vi "Pack Mag Dev Msg.vi"(11 "Compass Mag Dev":dbl) -> (3 "Set Mag Dev Message out":refnum<class "Set Mag Dev Message.lvclass">)   [LabVIEW 2015, in "Compass Instrument.lvlib"]
uses:
  Compass Instrument.lvlib
  Libraries/RDS Child Messages/Compass/Set Mag Dev Message.lvclass
  Libraries/RDS Framework/RDS Message ID.ctl
  Libraries/RDS Framework/RDS Message Class/RDS Message.lvclass/RDS Message.ctl
  Libraries/RDS Child Messages/Compass/Set Mag Dev Message.lvclass/Set Mag Dev Message.ctl
  Libraries/RDS Framework/RDS Message Class/RDS Message.lvclass
  Libraries/RDS Child Messages/RDS Child Messages.lvlib
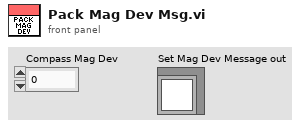
[diagram p1: front panel]
types:
  T1 = typedef "RDS Child Messages.lvlib/RDS Message ID.ctl" = enum16{"RDS Hello World", "String Message", "AIP_Status", "AIP_Command", "GPS_Data", "MCB_Command", "MCB_Status", "Compass_Data", "Depth_Data", "Battery_Data", "Contoller_State", "Set_Mag_Dev", "BTB_Shutdown", "State_Sample_Request", "State_Sample", "PID_Gains_Set", "Helm_Limiter_Set", "Helm_Heading_Command", "Helm_Steering_Command", "Helm_Status", "Controller_Message", "AIP_Set_Min_Depth", "Mission_Controller_State", "Mission_Upload", "Mission_Set_Op_and_Run", "Mission_Settings_Set"}
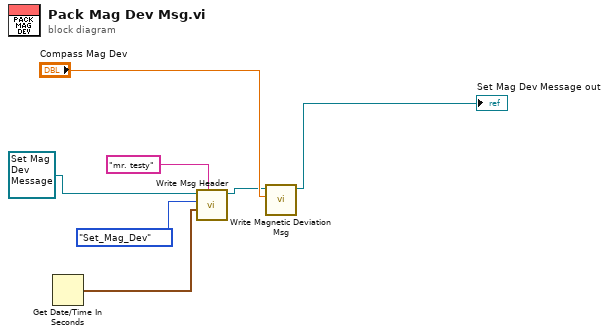
[diagram p0: block diagram]
diagram:
  n1 = Get Date/Time In Seconds() -> (seconds since 1Jan1904=w2:timestamp)
  n2 = call "Write Msg Header.vi"("Sender Name"="mr. testy", "Time Stamp"=w2, "Msg ID"=RDS_Message_ID."Set_Mag_Dev", "RDS Message in"=refnum<class "Set Mag Dev Message.lvclass"> refnum ("RDS Child Messages.lvlib:Set Mag Dev Message.lvclass")) -> ("RDS Message out"=w5:refnum<class "Set Mag Dev Message.lvclass">)  [unwired: 6 in, 1 out]
  n3 = call "Write Magnetic Deviation Msg.vi"("Magnetic Deviation"="Compass Mag Dev", "Set Mag Dev Message in"=w5) -> ("Set Mag Dev Message out"=→"Set Mag Dev Message out":refnum<class "Set Mag Dev Message.lvclass">)  [unwired: 8 in, 1 out]
